vi "myRIO_BRig_Host_TCP_parseCmd_BlockOrTrial__subunit.vi"(8 "input_arrayUnknown":i32[][](array[numeric]), 9 "input_idxUnknown":i32, 10 "input_countCmd":i32, 11 "input_strCmd":string) -> (0 "output_countTrial":i32, 1 "output_L/R":i32, 2 "output_iTrial":i32, 3 "output_iBlock":i32, 4 "output_idxUnknown":i32, 6 "output_arrayUnknown":i32[][](array[numeric]))   [LabVIEW 2014]
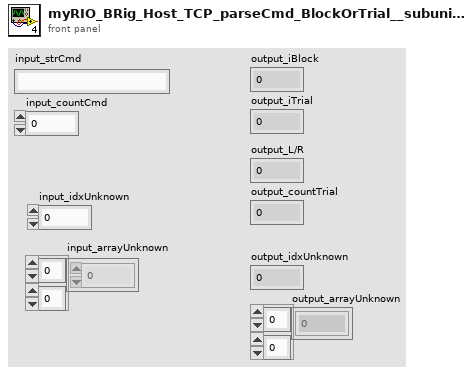
[diagram p1: front panel]
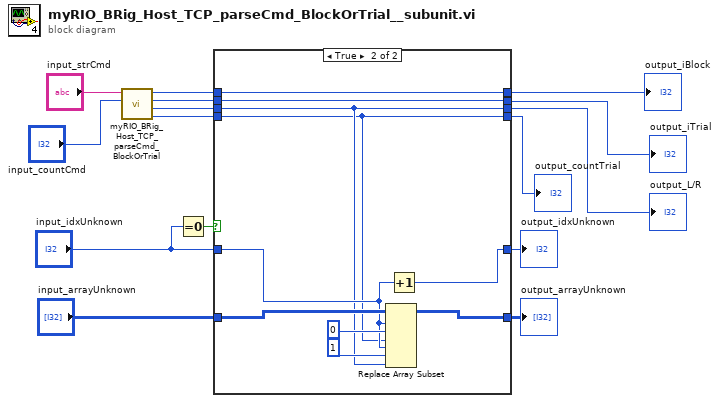
[diagram p0: block diagram]
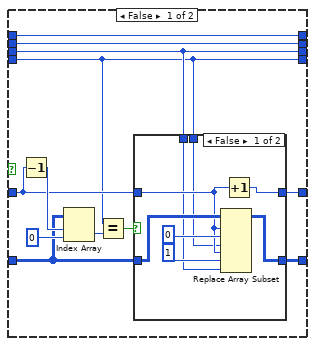
[diagram p2: hidden frame]
diagram:
  n1 = call "myRIO_BRig_Host_TCP_parseCmd_BlockOrTrial.vi"("input_countCmd"="input_countCmd", "input_strCmd"="input_strCmd") -> ("output_countTrial"=w9:i32, "output_L/R"=w10:i32, "output_iTrial"=w11:i32, "output_iBlock"=w12:i32)  [unwired: 6 in]
  n2 = Equal To 0?(x="input_idxUnknown") -> (x = 0?=w13:bool)
  n3 = case shown="True" w13 {
    tunnel: "input_idxUnknown" -> [w18 w44]
    tunnel: w12 -> [w23 w41]
    tunnel: w11 -> [w22 w40]
    tunnel: w10 -> [w17 w39]
    tunnel: w9 -> [w16 w38]
    tunnel: "input_arrayUnknown" -> [w21 w45]
    tunnel: [w20 w43] -> w2
    tunnel: [w19 w42] -> w3
    tunnel: [w23 w41] -> w7
    tunnel: [w22 w40] -> w6
    tunnel: [w17 w39] -> w5
    tunnel: [w16 w38] -> w4
    frame False {
      n4 = Decrement(x=w18) -> (x-1=w27:i32)
      n5 = Index Array(array=w21, index (row)=w27, index (col)=0 ("disabled index (col)")) -> (element=w25:i32)
      n6 = Equal?(x=w16, y=w25) -> (x = y?=w24:bool)
      n7 = case shown="False" w24 {
        tunnel: w21 -> [w33 w37]
        tunnel: [w28 w37] -> w20
        tunnel: [w31 w36] -> w19
        tunnel: w18 -> [w32 w36]
        tunnel: w17 -> [w30 _]
        tunnel: w16 -> [w29 _]
        frame False {
          n8 = Replace Array Subset(array=w33, new element #1=w29, index (row) #1=w32, index (col) #1=0 ("new element/subarray"), new element #2=w30, index (row) #2=w32, index (col) #2=1 ("new element/subarray")) -> (w28:i32[][])
          n9 = Increment(x=w32) -> (x+1=w31:i32)
        }
        frame True {
        }
      }
    }
    frame True {
      n10 = Replace Array Subset(array=w45, new element #1=w38, index (row) #1=w44, index (col) #1=0 ("new element/subarray"), new element #2=w39, index (row) #2=w44, index (col) #2=1 ("new element/subarray")) -> (w43:i32[][])
      n11 = Increment(x=w44) -> (x+1=w42:i32)
    }
  }
  "output_iBlock" <- w7
  "output_iTrial" <- w6
  "output_L/R" <- w5
  "output_countTrial" <- w4
  "output_idxUnknown" <- w3
  "output_arrayUnknown" <- w2
